vi "Trend-algo.vi"(5 "LSL":dbl, 7 "USL":dbl, 8 "error in (no error)":errorcluster, 10 "ReducedOutputData":dbl[][](array[numeric])) -> (0 "error out":errorcluster, 2 "OutputData-Trend":dbl[][](array[numeric]))   [LabVIEW 2019, in "Zen Analytics.lvlib" / "Zen Analytics.lvclass"]
uses:
  Zen Analytics.lvclass
panel:
  out "Waveform Graph":dbl[][](graph)
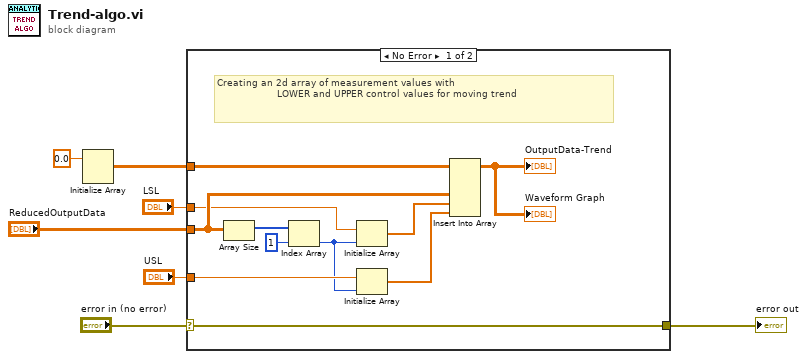
[diagram p0: block diagram]
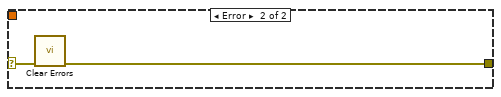
[diagram p2: hidden frame]
diagram:
  n1 = Initialize Array "Initialize Array"(0.0 ("element")) -> (w4:dbl[][])  [unwired: 2 in]
  n2 = case shown="No Error" "error in (no error)" {
    selector: "error in (no error)" -> [w15 w20]
    tunnel: [w15 w19] -> w1
    tunnel: "ReducedOutputData" -> [w13 _]
    tunnel: "LSL" -> [w12 _]
    tunnel: "USL" -> [w10 _]
    tunnel: w4 -> [w18 _]
    frame No Error {
      # "Creating an 2d array of measurement values with \n                    LOWER and UPPER control values for moving trend"
      n3 = Array Size(array=w13) -> (size(s)=w17:i32[])
      n4 = Index Array(array=w17, index=1) -> (element=w8:i32)
      n5 = Initialize Array(w12, w8) -> (w11:dbl[])
      n6 = Initialize Array(w10, w8) -> (w9:dbl[])
      n7 = Insert Into Array(array=w18, new element #1=w13, new element #2=w11, new element #3=w9) -> (→"OutputData-Trend" →"Waveform Graph":dbl[][])  [unwired: 2 in]
    }
    frame Error {
      n8 = call <vilib>:"Clear Errors.vi"("error in (no error)"=w20) -> ("error out"=w19:errorcluster)  [unwired: 5 in, 1 out]
    }
  }
  "error out" <- w1
